vi "Verify by Setpoint percentage - Alternate v2.vi"(5 "Mode":enum16{"Band", "UpperLimit", "LowerLimit"}(ring), 7 "Settings":T1={"AnalogBand Enable"=FALSE, "Fault(%)"=1.0, "Warning(%)"=5.0, "Stabilization time (ms)"=2000} {"Fault(%)" format="%#_g%%"; "Warning(%)" format="%#_g%%"}, 10 "Actual Value":dbl, 11 "Set Point":dbl) -> (1 "InRange?":bool, 2 "Fault?":bool, 3 "Warning?":bool)   [LabVIEW 2017]
doc: "Developed by Kevin Thompson\nkevin@thompsonengineering.net\n\nCopyright 2018-2020\nThompson Engineering, LLC"
uses:
  <vilib>/TELLC/Misc Utilities/AB Settings--cluster.ctl
  <userlib>/_OpenG.lib/comparison/comparison.llb/DBL Changed__ogtk.vi
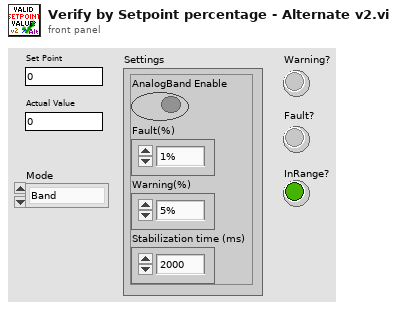
[diagram p1: front panel]
types:
  T1 = typedef "AB Settings--cluster.ctl" = cluster{"AnalogBand Enable":bool, "Fault(%)":dbl, "Warning(%)":dbl, "Stabilization time (ms)":u32}
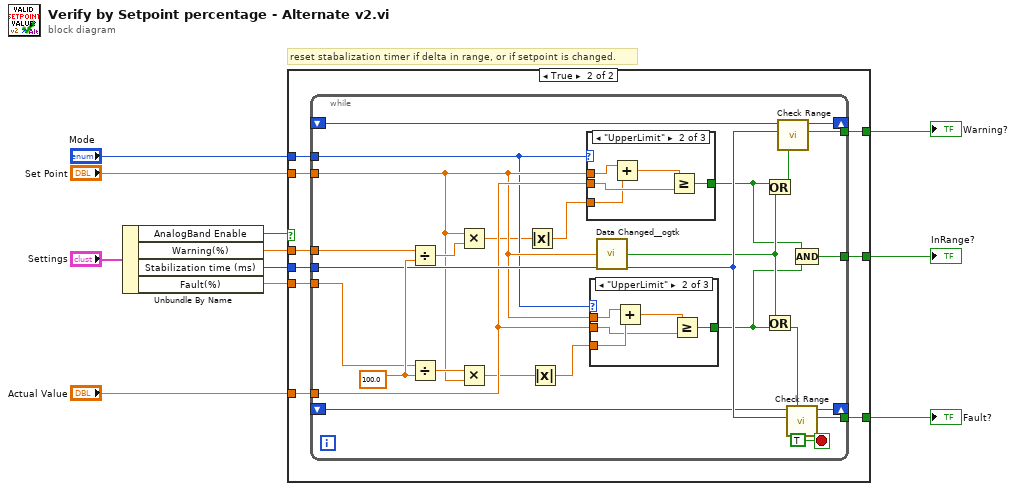
[diagram p0: block diagram]
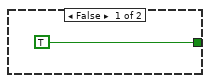
[diagram p2: hidden frame]
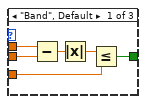
[diagram p3: hidden frame]
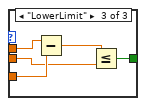
[diagram p4: hidden frame]
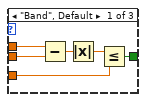
[diagram p5: hidden frame]
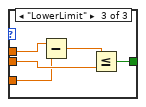
[diagram p6: hidden frame]
diagram:
  # "reset stabalization timer if delta in range, or if setpoint is changed."
  n1 = Unbundle By Name("Settings") -> ("AnalogBand Enable"=w3:bool, "Warning(%)"=w10:dbl, "Stabilization time (ms)"=w6:u32, "Fault(%)"=w7:dbl)
  n2 = case shown="True" w3 {
    tunnel: w10 -> [_ w21]
    tunnel: "Set Point" -> [_ w20]
    tunnel: "Actual Value" -> [_ w19]
    tunnel: w7 -> [_ w18]
    tunnel: w6 -> [_ w17]
    tunnel: [_ w16] -> w5
    tunnel: [_ w15] -> w4
    tunnel: [TRUE w14] -> w2
    tunnel: "Mode" -> [_ w13]
    frame False {
    }
    frame True {
      n3 = while {
        tunnel: w21 -> [w46]
        tunnel: w20 -> [w32]
        tunnel: w19 -> [w34]
        tunnel: w18 -> [w42]
        tunnel: w17 -> [w39]
        shift-right: [w41] -> _
        shift-left: _ -> [w40]
        tunnel: [w35] -> w16
        tunnel: [w38] -> w15
        shift-right: [w37] -> _
        shift-left: _ -> [w36]
        tunnel: [w27] -> w14
        tunnel: w13 -> [w26]
        stop <- TRUE stop-if-true
        w45 = 100.0 ("y")
        n4 = Divide(x=w46, y=w45) -> (x/y=w44:dbl)
        n5 = Divide(x=w42, y=w45) -> (x/y=w47:dbl)
        n6 = Multiply(x=w32, y=w44) -> (x*y=w24:dbl)
        n7 = Multiply(x=w47, y=w32) -> (x*y=w25:dbl)
        n8 = Absolute Value(x=w24) -> (abs(x)=w22:dbl)
        n9 = Absolute Value(x=w25) -> (abs(x)=w23:dbl)
        n10 = case shown="\"UpperLimit\"" w26 {
          tunnel: w34 -> [w67 w72 w77]
          tunnel: w32 -> [w66 w71 w76]
          tunnel: [w65 w73 w78] -> w28
          tunnel: w22 -> [w64 w70 w75]
          frame "Band", Default {
            n11 = Subtract(x=w66, y=w67) -> (x-y=w68:dbl)
            n12 = Absolute Value(x=w68) -> (abs(x)=w69:dbl)
            n13 = Less Or Equal?(x=w69, y=w64) -> (x <= y?=w65:bool)
          }
          frame "UpperLimit" {
            n14 = Add(x=w71, y=w70) -> (x+y=w74:dbl)
            n15 = Greater Or Equal?(x=w74, y=w72) -> (x >= y?=w73:bool)
          }
          frame "LowerLimit" {
            n16 = Subtract(x=w76, y=w75) -> (x-y=w79:dbl)
            n17 = Less Or Equal?(x=w79, y=w77) -> (x <= y?=w78:bool)
          }
        }
        n18 = case shown="\"UpperLimit\"" w26 {
          tunnel: w34 -> [w51 w54 w59]
          tunnel: w32 -> [w50 w57 w62]
          tunnel: [w49 w58 w63] -> w29
          tunnel: w23 -> [w48 w56 w61]
          frame "Band", Default {
            n19 = Subtract(x=w50, y=w51) -> (x-y=w53:dbl)
            n20 = Absolute Value(x=w53) -> (abs(x)=w52:dbl)
            n21 = Less Or Equal?(x=w52, y=w48) -> (x <= y?=w49:bool)
          }
          frame "UpperLimit" {
            n22 = Add(x=w57, y=w56) -> (x+y=w55:dbl)
            n23 = Greater Or Equal?(x=w55, y=w54) -> (x >= y?=w58:bool)
          }
          frame "LowerLimit" {
            n24 = Subtract(x=w62, y=w61) -> (x-y=w60:dbl)
            n25 = Less Or Equal?(x=w60, y=w59) -> (x <= y?=w63:bool)
          }
        }
        n26 = call-poly <userlib>:"Data Changed__ogtk.vi"("DBL"=w32) -> ("Changed"=w31:bool)
        n27 = Or(x=w28, y=w31) -> (x .or. y?=w30:bool)
        n28 = Or(x=w31, y=w29) -> (x .or. y?=w33:bool)
        n29 = call <vilib>:"Check Range.vi"("approx = ?"=w30, "Stabilization time (ms)"=w39, "millisecond timer value"=w40) -> ("Valid"=w35:bool, "elapsed"=w41:u32)  [unwired: 7 in]
        n30 = call <vilib>:"Check Range.vi"("approx = ?"=w33, "Stabilization time (ms)"=w39, "millisecond timer value"=w36) -> ("Valid"=w38:bool, "elapsed"=w37:u32)  [unwired: 7 in]
        n31 = Compound Arithmetic op=AND(w28, w29) -> (w27:bool)
      }
    }
  }
  "Fault?" <- w4
  "Warning?" <- w5
  "InRange?" <- w2
